vi "Async.Read Data from HW.vi"(8 "error in":errorcluster, 11 "Async in":refnum<class "VS Inline Async API.lvclass">) -> (0 "error out":errorcluster, 3 "Async out":refnum<class "VS Inline Async API.lvclass">)   [LabVIEW 2015, in "VS Inline Async API.lvlib" / "VS Inline Async API.lvclass"]
uses:
  VS Inline Async API.lvclass
  VS Inline Async API.lvclass/VS Inline Async API.ctl
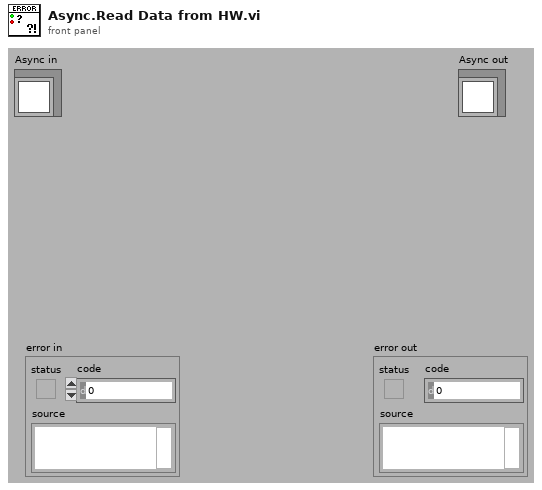
[diagram p1: front panel]
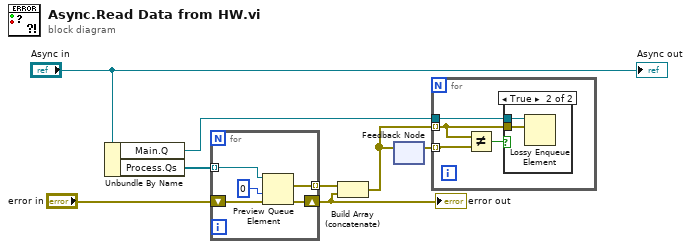
[diagram p0: block diagram]
diagram:
  n1 = Unbundle By Name("Async in") -> ("Main.Q"=w4:refnum<queue>, "Process.Qs"=w3:refnum<queue>[])
  n2 = for {
    tunnel: w3 -> [w12] mode=indexing
    shift-right: [w10] -> w2
    shift-left: "error in" -> [w13]
    tunnel: [w9] -> w7 mode=indexing
    n3 = Preview Queue Element(queue=w12, timeout in ms (-1)=0, error in (no error)=w13) -> (element=w9:errorcluster, error out=w10:errorcluster)  [unwired: 2 out]
  }
  "error out" <- w2
  n4 = Build Array (concatenate)(w7, w2) -> (w5:errorcluster[])
  n5 = feedback #1() -> (w6:errorcluster[])  [unwired: 1 in]
  n6 = feedback-in #1(w5) -> ()
  n7 = for {
    tunnel: w6 -> [w17] mode=indexing
    tunnel: w4 -> [w16]
    tunnel: w5 -> [w15] mode=indexing
    n8 = Not Equal?(x=w15, y=w17) -> (x != y?=w14:bool)
    n9 = case shown="True" w14 {
      tunnel: w16 -> [_ w19]
      tunnel: w15 -> [_ w18]
      frame False {
      }
      frame True {
        n10 = Lossy Enqueue Element(queue=w19, element=w18) -> ()  [unwired: 1 in, 4 out]
      }
    }
  }
  "Async out" <- "Async in"
